vi "EOL CAN_Get_Motor_Voltage.vi"(8 "Error in":errorcluster, 10 "Read Session in":refnum<k21>, 11 "Write Session in":refnum<k21>) -> (0 "Error out":errorcluster, 1 "Motor Voltage":dbl, 2 "TxRx Data":string[][](array[string]), 3 "Response Good?":bool)   [LabVIEW 2012]
uses:
  <vilib>/xnet/xnet.llb/XNET Frame Type CAN.ctl
  <vilib>/xnet/xnet.llb/XNET Frame CAN.ctl
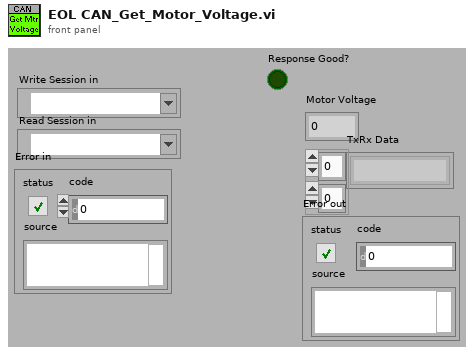
[diagram p1: front panel]
types:
  T1 = typedef "XNET Frame CAN.ctl" = cluster{"timestamp":timestamp, "payload":u8[], "identifier":u32, "type":T2, "extended?":bool, "echo?":bool}
  T2 = typedef "XNET Frame Type CAN.ctl" = u8
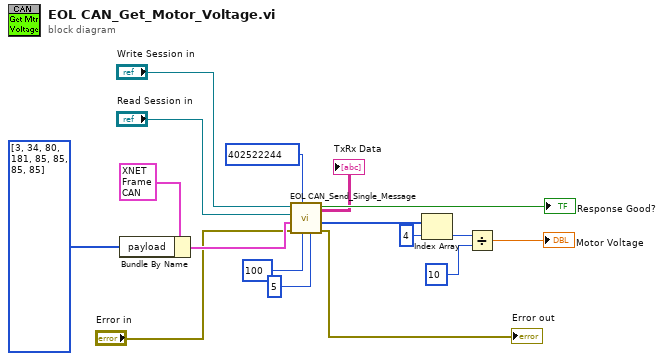
[diagram p0: block diagram]
diagram:
  n1 = Bundle By Name(cluster=T1 {"timestamp"=timestamp(0 s since 1904-01-01), "payload"=[2, 39, 3, 85, 85, 85, 85, 85], "identifier"=402391172, "type"=8, "extended?"=TRUE, "echo?"=FALSE} ("Tx CAN frame"), "payload"=u8[] [3, 34, 80, 181, 85, 85, 85, 85] ("Transmit Data")) -> (w7:T1)
  n2 = call "EOL CAN_Send_Single_Message.vi"("Retries"=5, "Msg Wait Time"=u32 100, "Rx Arbitration Id"=u32 402522244, "Error in"="Error in", "Tx CAN frame"=w7, "Read Session in"="Read Session in", "Write Session in"="Write Session in") -> ("Error out"=→"Error out":errorcluster, "Rx Message"=w13:u8[], "Response Good?"=→"Response Good?":bool, "TxRx Data"=→"TxRx Data":string[][])  [unwired: 1 out]
  n3 = Index Array(array=w13, index=4) -> (element=w15:u8)
  n4 = Divide(x=w15, y=u8 10) -> (x/y=→"Motor Voltage":dbl)
